vi "DBM Start.vi"(8 "에러 입력(에러 없음)":errorcluster, 11 "추가된 배열":refnum<vi>[](array[refnum])) -> (0 "에러 출력":errorcluster, 2 "사용자 이벤트 - 정지":refnum<user-event>, 3 "큐 출력":refnum<queue>, 4 "dup path":path, 5 "이벤트 등록 참조 번호 출력":refnum<event-registration>, 6 "배열":string[](array[string]))   [LabVIEW 2020]
uses:
  Controls/Message Cluster.ctl
  Controls/Cmd_File path.ctl
  <vilib>/Utility/sysdir.llb/System Directory Type.ctl
  Controls/Cmd_File Type.ctl
  Variables/Global_Constant.vi
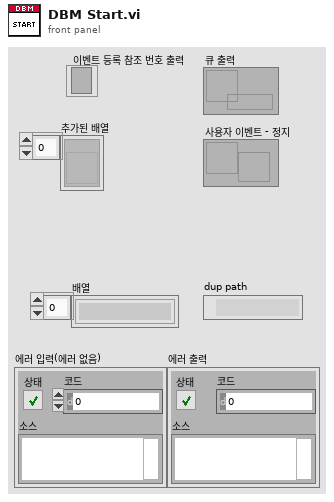
[diagram p1: front panel]
types:
  T1 = typedef "Cmd_File Type.ctl" = enum16{"엑셀", "엑셀(2003)", "텍스트", "설정", "2진", "VI", "CSV", "LOG", "폴더"}
  T2 = typedef "System Directory Type.ctl" = i32
  T3 = typedef "Cmd_File path.ctl" = enum16{"에러로그", "데이터파일경로", "성적서원본", "지난성적서", "Data Files", "경로생성", "Updater", "Template", "설정파일경로", "FTP Upload", "Update 경로", "어플리케이션"}
  T4 = enum32{"invalid app kind", "Development System", "Run Time System", "Student Edition", "Embedded LabVIEW", "Evaluation", "Custom"}
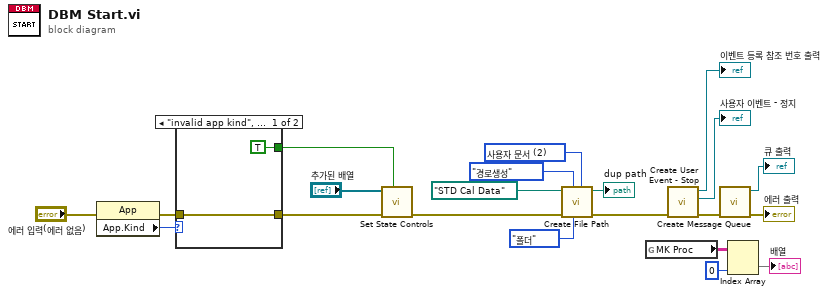
[diagram p0: block diagram]
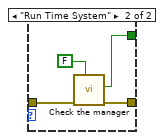
[diagram p2: hidden frame]
diagram:
  w8 = T2 2 items=["사용자 홈"=0, "사용자 데스크탑"=1, "사용자 문서"=2, "사용자 어플리케이션 데이터"=3, "사용자 환경"=4, "사용자 임시"=5, "퍼블릭 문서"=6, "퍼블릭 어플리케이션 데이터"=7, "퍼블릭 환경"=8, "퍼블릭 캐시"=13, "시스템 코어 라이브러리"=9, "시스템 설치된 라이브러리"=10, "어플리케이션 파일"=11, "부팅 볼륨 루트"=12] ("system directory type")
  n1 = property class="App"(error in="에러 입력(에러 없음)") -> (error out=w2:errorcluster, "App.Kind"=w1:T4)  [unwired: 1 in, 1 out]
  n2 = case shown="\"invalid app kind\", 기본" w1 {
    tunnel: w2 -> [w23 w27]
    tunnel: [w23 w26] -> w5
    tunnel: [TRUE ("OK?") w25] -> w4
    frame "invalid app kind", Default {
    }
    frame "Run Time System" {
      n3 = call "Check the manager.vi"("불리언"=FALSE, "error in (no error)"=w27) -> ("error out"=w26:errorcluster, "OK?"=w25:bool)  [unwired: 8 in]
    }
  }
  n4 = call "Set State Controls.vi"("활성화 (F)"=w4, "error in (no error)"=w5, "컨트롤 참조 배열 in"="추가된 배열") -> ("error out"=w10:errorcluster)  [unwired: 7 in, 1 out]
  n5 = call "Create File Path.vi"("system directory type"=w8, "파일타입"=Cmd_File_Type."폴더", "항목"=Cmd_File_path."경로생성", "에러 입력"=w10, "폴더명 in"=path "STD Cal Data" ("STD File Path")) -> ("error out"=w9:errorcluster, "파일경로"=→"dup path":path)  [unwired: 3 in, 2 out]
  n6 = global read "Global_Constant.vi" "MK Proc"() -> (w15:string[][])
  n7 = call "Create User Event - Stop.vi"("에러 입력(에러 없음)"=w9) -> ("에러 출력"=w19:errorcluster, "사용자 이벤트 - 정지"=→"사용자 이벤트 - 정지":refnum<user-event>, "이벤트 등록 참조 번호 출력"=→"이벤트 등록 참조 번호 출력":refnum<event-registration>)  [unwired: 8 in]
  n8 = call "Create Message Queue.vi"("에러 입력(에러 없음)"=w19) -> ("에러 출력"=→"에러 출력":errorcluster, "큐 출력"=→"큐 출력":refnum<queue>)  [unwired: 9 in]
  n9 = Index Array(array=w15, index (col)=0 ("비활성화된 인덱스 (열)")) -> (element=→"배열":string[])  [unwired: 1 in]
